vi "delete_collection.vi"(0 "vector_qdrant in":refnum<class "vector_qdrant.lvclass">, 5 "collection_name":string, 11 "error in (no error)":errorcluster) -> (4 "vector_qdrant out":refnum<class "vector_qdrant.lvclass">, 15 "error out":errorcluster)   [LabVIEW 2020, in "vector_qdrant.lvclass"]
uses:
  vector_qdrant.lvclass
  vector_qdrant.lvclass/vector_qdrant.ctl
  <vilib>/httpClient/LabVIEWHTTPClient.lvlib
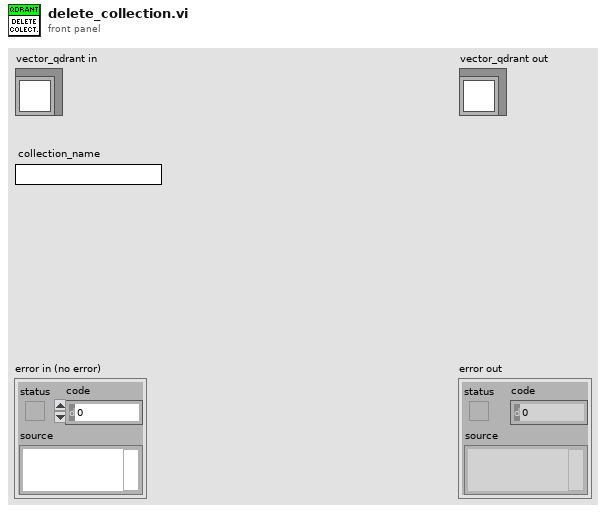
[diagram p1: front panel]
types:
  T1 = typedef "LabVIEWHTTPClient.lvlib/ClientHandle.ctl" = refnum<k1>
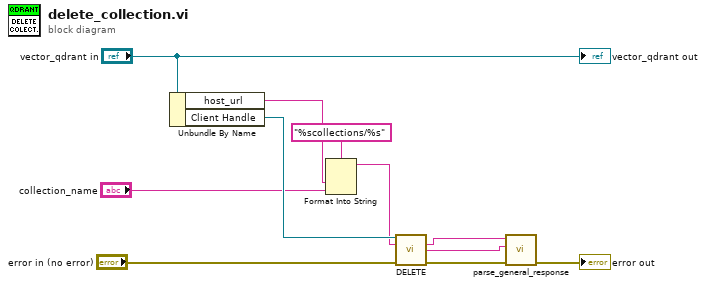
[diagram p0: block diagram]
diagram:
  n1 = Unbundle By Name("vector_qdrant in") -> ("host_url"=w7:string, "Client Handle"=w9:T1)
  n2 = Format Into String(format string="%scollections/%s", w7, "collection_name") -> (resulting string=w5:string)  [unwired: 2 in, 1 out]
  n3 = call <vilib>:"DELETE.vi"("client handle"=w9, "url"=w5, "error in (no error)"="error in (no error)") -> ("headers"=w2:string, "body"=w1:string, "error out"=w4:errorcluster)  [unwired: 9 in, 1 out]
  n4 = call "parse_general_response.vi"("error in (no error)"=w4, "body"=w1, "headers"=w2) -> ("error out"=→"error out":errorcluster)  [unwired: 8 in]
  "vector_qdrant out" <- "vector_qdrant in"
